vi "test_Create MetaData Channel_array type cast.vi"(8 "error in (no error)":errorcluster, 11 "TestCase in":refnum<class "Instrument Addon Scripting API Channels Unit Tests.lvclass">) -> (0 "error out":errorcluster, 3 "TestCase out":refnum<class "Instrument Addon Scripting API Channels Unit Tests.lvclass">)   [LabVIEW 2018, in "Instrument Addon Scripting API Channels Unit Tests.lvclass"]
uses:
  Instrument Addon Scripting API Channels Unit Tests.lvclass
  <vilib>/addons/_JKI Toolkits/VI Tester/TestCase.llb/TestCase.lvclass
  Instrument Addon Scripting API Test Assets/Instrument Addon Scripting API Test Assets.lvclass
  <vilib>/NI Veristand/Custom Device Tools/Custom Device Utility Library/Custom Device Utility Library.lvlib
  Addon/Addon Shared/SubVIs/Constants.vi
  Addon/Addon Shared/Instrument Addon Shared.lvlib
  Addon/Addon Shared/Types/FG Control.ctl
  APIs/Scripting API/TypeDefs/Array Element.ctl
  APIs/Scripting API/Instrument Addon Scripting API.lvlib
  Addon/Addon Shared/Types/Type Cast Type.ctl
  Addon/Addon Shared/Types/Endian.ctl
  APIs/Scripting API/TypeDefs/Array Type Cast Settings.ctl
  <vilib>/NI Veristand/Custom Device Tools/Custom Device Utility Library/NI VeriStand - Search for Item by Name.vi
  <vilib>/NI Veristand/Custom Device Tools/Custom Device Utility Library/NI VeriStand - Search for Item by GUID.vi
  C:/Program Files (x86)/National Instruments/LabVIEW 2018/vi.lib/addons/_JKI Toolkits/VI Tester/TestCase.llb/TestCase.lvclass
  APIs/Scripting API/Channels/Create MetaData Channel - Array - Type Cast.vi
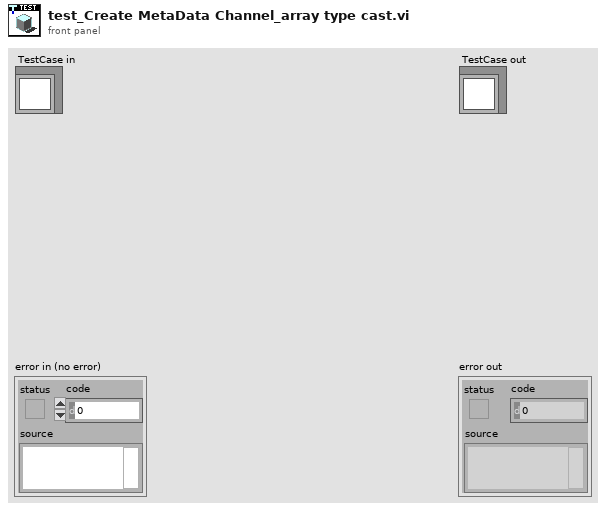
[diagram p1: front panel]
types:
  T1 = typedef "Instrument Addon Shared.lvlib/FG Control.ctl" = enum16{"Get", "Set"}
  T2 = typedef "Instrument Addon Scripting API.lvlib/Array Type Cast Settings.ctl" = cluster{"Elements":T3[], "Type":T4, "Endian":T5, "Delimiter":string}
  T3 = typedef "Instrument Addon Scripting API.lvlib/Array Element.ctl" = cluster{"Name":string, "Default Value":dbl, "Units":string}
  T4 = typedef "Instrument Addon Shared.lvlib/Type Cast Type.ctl" = enum16{"DBL", "SGL", "U64", "U32", "U16", "U8", "I64", "I32", "I16", "I8"}
  T5 = typedef "Instrument Addon Shared.lvlib/Endian.ctl" = enum16{"Native", "Little", "Big"}
  T6 = typedef "Custom Device API.lvlib/Custom Device Item Ref.ctl" = u64
  T7 = typedef "Instrument Addon Shared.lvlib/MetaData Parameters.ctl" = cluster{"Data Type":T8, "Channel Type":T9, "List":string[], "Format String":string, "Type":T4, "Delimiter":string, "Endian":T5}
  T8 = typedef "Instrument Addon Shared.lvlib/Protocol Data Type.ctl" = enum16{"Single Channel", "Array"}
  T9 = typedef "Instrument Addon Shared.lvlib/Metadata Channel Type.ctl" = enum16{"Enumerated List", "Format", "Type Cast"}
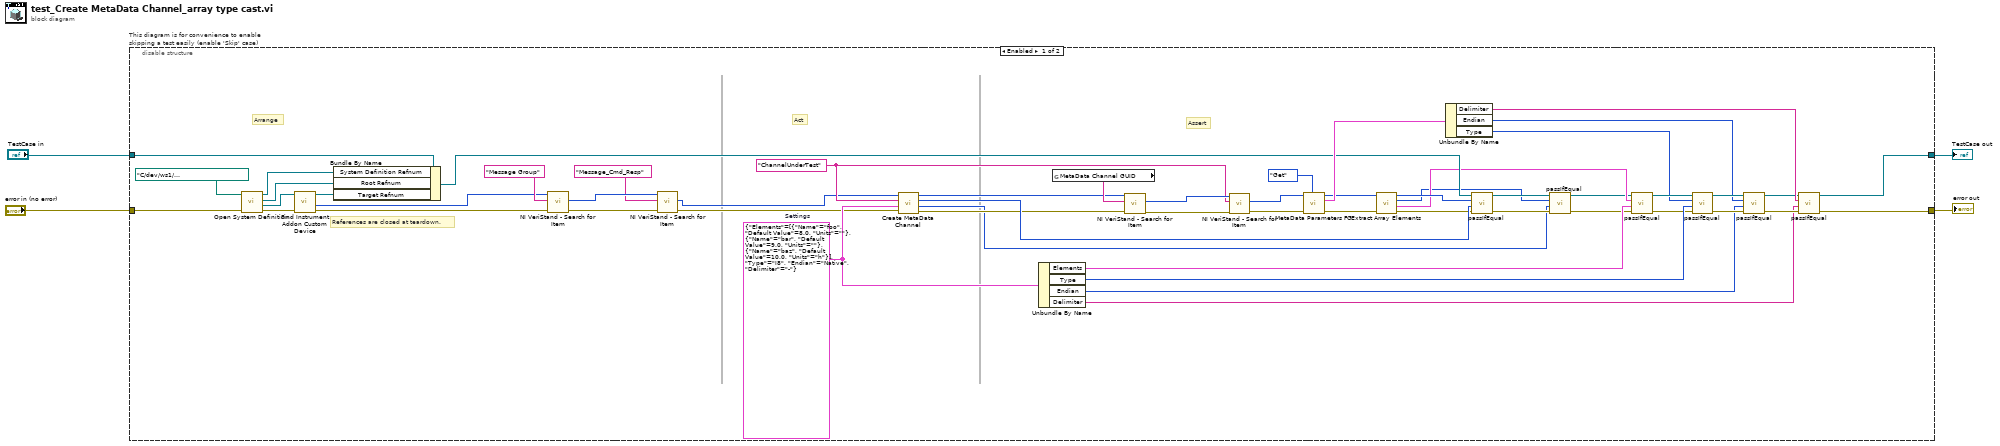
[diagram p0: block diagram]
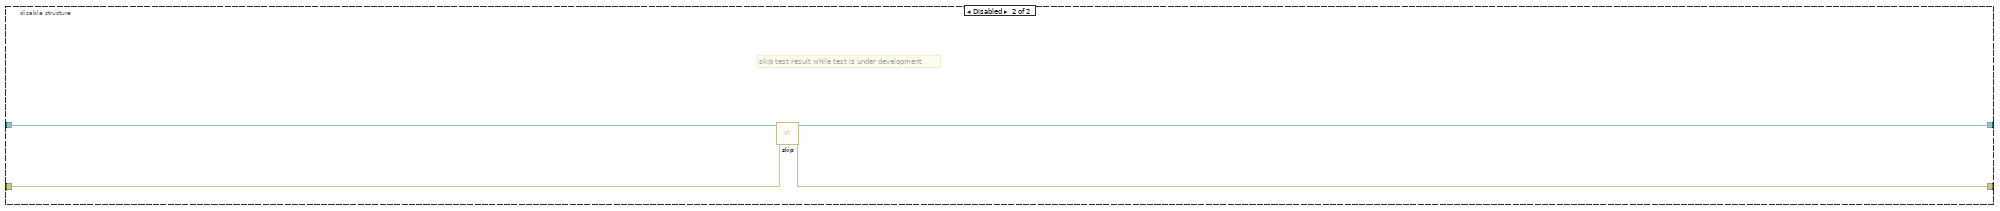
[diagram p2: hidden frame]
diagram:
  n1 = disable-structure "This diagram is for convenience to enable skipping a test easily (enable 'Skip' case)" shown="Enabled" {
    disable-tunnel: "TestCase in" -> [w43 w63]
    disable-tunnel: [w37 w61] -> w1
    disable-tunnel: [w36 w62] -> w3
    disable-tunnel: "error in (no error)" -> [w59 w60]
    frame Enabled {
      w28 = T2 {"Elements"=[{"Name"="foo", "Default Value"=8.0, "Units"=""}, {"Name"="bar", "Default Value"=9.0, "Units"=""}, {"Name"="baz", "Default Value"=10.0, "Units"="h"}], "Type"=enum."I8", "Endian"=enum."Native", "Delimiter"="-"}  # Settings
      w42 = "ChannelUnderTest" ("Name")
      # "References are closed at teardown."
      # "Assert"
      # "Act"
      # "Arrange"
      n2 = call "Open System Definition.vi"("error in (no error)"=w59, "System Definition File"=path "C:/dev/ws1/niveristand-instrument-addon-custom-device/Source/Tests/Unit Tests/Scripting API/Instrument Addon Scripting API Channels Unit Tests/Assets/MetaData Channels/IACD_channels.nivssdf") -> ("error out"=w57:errorcluster, "Target Refnum"=w58:refnum<k24>, "Root Refnum"=w46:refnum<k24>, "System Definition Refnum"=w45:refnum<k24>)  [unwired: 6 in]
      n3 = call "Find Instrument Addon Custom Device.vi"("error in"=w57, "target in"=w58) -> ("error out"=w14:errorcluster, "NodeID"=w15:u64, "target out"=w47:refnum<k24>)  [unwired: 7 in]
      n4 = Bundle By Name(cluster=w43, "System Definition Refnum"=w45, "Root Refnum"=w46, "Target Refnum"=w47) -> (w44:refnum<class "Instrument Addon Scripting API Channels Unit Tests.lvclass">)
      n5 = call-poly <vilib>:"NI VeriStand - Search for Item.vi"("error in"=w14, "Item Name"="Message Group", "Section Ref in"=w15) -> ("error out"=w16:errorcluster, "Item Ref"=w18:T6)  [unwired: 5 in, 2 out]
      n6 = call-poly <vilib>:"NI VeriStand - Search for Item.vi"("error in"=w16, "Item Name"="Message_Cmd_Resp", "Section Ref in"=w18) -> ("error out"=w12:errorcluster, "Item Ref"=w13:T6)  [unwired: 5 in, 2 out]
      n7 = call-poly "Create MetaData Channel.vi"("Error In"=w12, "Settings"=w28, "Name"=w42, "Message Refnum In"=w13) -> ("Error Out"=w39:errorcluster, "Channel Refnums"=w5:T6[], "Array Refnum"=w40:T6, "Message Refnum Out"=w41:T6)  [unwired: 4 in]
      n8 = Unbundle By Name(w28) -> ("Elements"=w33:T3[], "Type"=w48:T4, "Endian"=w23:T5, "Delimiter"=w20:string)
      n9 = global read "Constants.vi" "MetaData Channel GUID"() -> (w55:string)
      n10 = call-poly <vilib>:"NI VeriStand - Search for Item.vi"("error in"=w39, "Item GUID"=w55, "Section Ref in"=w41) -> ("error out"=w53:errorcluster, "Item Ref"=w54:T6)  [unwired: 5 in, 2 out]
      n11 = call-poly <vilib>:"NI VeriStand - Search for Item.vi"("error in"=w53, "Item Name"=w42, "Section Ref in"=w54) -> ("error out"=w52:errorcluster, "Item Ref"=w51:T6)  [unwired: 5 in, 2 out]
      n12 = call "MetaData Parameters FG.vi"("Action"=FG_Control."Get", "error in (no error)"=w52, "Item Ref in"=w51) -> ("error out"=w32:errorcluster, "MetaData Parameters"=w49:T7, "Item Ref out"=w31:T6)  [unwired: 6 in]
      n13 = call "Extract Array Elements.vi"("error in (no error)"=w32, "array reference in"=w31) -> ("error out"=w30:errorcluster, "elements"=w11:T3[], "channel refnums"=w6:T6[], "array reference out"=w29:T6)  [unwired: 6 in]
      n14 = Unbundle By Name(w49) -> ("Delimiter"=w38:string, "Endian"=w21:T5, "Type"=w22:T4)
      n15 = call-dynamic "passIfEqual.vi"("error in (no error)"=w30, "y"=w40, "x"=w29, "TestCase in"=w44) -> ("error out"=w9:errorcluster, "TestCase out"=w10:refnum<class "Instrument Addon Scripting API Channels Unit Tests.lvclass">)  [unwired: 6 in]
      n16 = call-dynamic "passIfEqual.vi"("error in (no error)"=w9, "y"=w5, "x"=w6, "TestCase in"=w10) -> ("error out"=w7:errorcluster, "TestCase out"=w8:refnum<class "Instrument Addon Scripting API Channels Unit Tests.lvclass">)  [unwired: 6 in]
      n17 = call-dynamic "passIfEqual.vi"("error in (no error)"=w7, "y"=w33, "x"=w11, "TestCase in"=w8) -> ("error out"=w34:errorcluster, "TestCase out"=w35:refnum<class "Instrument Addon Scripting API Channels Unit Tests.lvclass">)  [unwired: 6 in]
      n18 = call-dynamic "passIfEqual.vi"("error in (no error)"=w34, "y"=w48, "x"=w22, "TestCase in"=w35) -> ("error out"=w26:errorcluster, "TestCase out"=w27:refnum<class "Instrument Addon Scripting API Channels Unit Tests.lvclass">)  [unwired: 6 in]
      n19 = call-dynamic "passIfEqual.vi"("error in (no error)"=w26, "y"=w23, "x"=w21, "TestCase in"=w27) -> ("error out"=w24:errorcluster, "TestCase out"=w25:refnum<class "Instrument Addon Scripting API Channels Unit Tests.lvclass">)  [unwired: 6 in]
      n20 = call-dynamic "passIfEqual.vi"("error in (no error)"=w24, "y"=w20, "x"=w38, "TestCase in"=w25) -> ("error out"=w36:errorcluster, "TestCase out"=w37:refnum<class "Instrument Addon Scripting API Channels Unit Tests.lvclass">)  [unwired: 6 in]
    }
    frame Disabled {
      # "skip test result while test is under development"
      n21 = call <vilib>:"skip.vi"("error in (no error)"=w60, "TestCase in"=w63) -> ("error out"=w62:errorcluster, "TestCase out"=w61:refnum<class "Instrument Addon Scripting API Channels Unit Tests.lvclass">)  [unwired: 8 in]
    }
  }
  "error out" <- w3
  "TestCase out" <- w1
